vi "Check - Methods Exist.vi"(10 "QControl Class Name":string, 11 "New Class Root Path":path) -> (0 "error out":errorcluster)   [LabVIEW 2015, in "QControl Creation.lvclass"]
doc: "<b> </b> <b> </b>\n©2016 Q Software Innovations, LLC (QSI)\nwritten by Quentin Alldredge\nproduced in LabVIEW 2015\n\nsupport@qsoftwareinnovations.com\nwww.qsoftwareinnovations.com\n\nAll rights reserved.\n\nRedistribution and use in source and binary forms, with or without modification, are permitted provided that the following conditions are met:\n\n * Redistributions of source code must retain the above copyright notice, this list of conditions and the following disclaimer.\n * Redistributions in binary form must reproduce the above copyright notice, this list of conditions and the following disclaimer in the documentation and/or other materials provided with the distribution.\n * Neither the name of Q Software Innovations, LLC. nor the names of its contributors may be used to endorse or promote products derived from this software without specific prior written permission.\n\nTHIS SOFTWARE IS PROVIDED BY THE COPYRIGHT HOLDERS AND CONTRIBUTORS \"AS IS\" AND ANY EXPRESS OR IMPLIED WARRANTIES, INCLUDING, BUT NOT LIMITED TO, THE IMPLIED WARRANTIES OF MERCHANTABILITY AND FITNESS FOR A PARTICULAR PURPOSE ARE DISCLAIMED. IN NO EVENT SHALL THE COPYRIGHT OWNER OR CONTRIBUTORS BE LIABLE FOR ANY DIRECT, INDIRECT, INCIDENTAL, SPECIAL, EXEMPLARY, OR CONSEQUENTIAL DAMAGES (INCLUDING, BUT NOT LIMITED TO, PROCUREMENT OF SUBSTITUTE GOODS OR SERVICES; LOSS OF USE, DATA, OR PROFITS; OR BUSINESS INTERRUPTION) HOWEVER CAUSED AND ON ANY THEORY OF LIABILITY, WHETHER IN CONTRACT, STRICT LIABILITY, OR TORT (INCLUDING NEGLIGENCE OR OTHERWISE) ARISING IN ANY WAY OUT OF THE USE OF THIS SOFTWARE, EVEN IF ADVISED OF THE POSSIBILITY OF SUCH DAMAGE."
uses:
  QControl Creation.lvclass
  Template/Template.lvclass
  <vilib>/ErrorRing/Error Ring.xnode
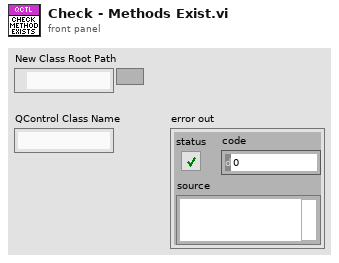
[diagram p1: front panel]
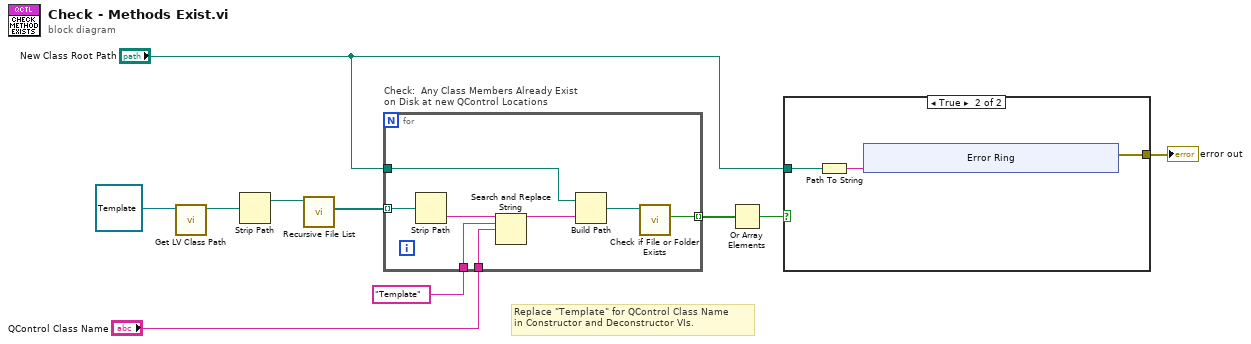
[diagram p0: block diagram]
diagram:
  # "Replace \"Template\" for QControl Class Name\nin Constructor and Deconstructor VIs."
  n1 = call <vilib>:"Get LV Class Path.vi"("object"=refnum<class "Template.lvclass"> refnum ("Template")) -> ("class path"=w8:path)  [unwired: 9 in, 1 out]
  n2 = Strip Path(path=w8) -> (stripped path=w9:path)  [unwired: 1 out]
  n3 = call <vilib>:"Recursive File List.vi"("Folder Path"=w9) -> ("All Files in Dir"=w10:path[])  [unwired: 6 in, 4 out]
  n4 = for "Check:  Any Class Members Already Exist \non Disk at new QControl Locations" {
    tunnel: w10 -> [w15] mode=indexing
    tunnel: "New Class Root Path" -> [w18]
    tunnel: [w17] -> w6 mode=indexing
    tunnel: "Template" ("search string") -> [w13]
    tunnel: "QControl Class Name" -> [w12]
    n5 = Strip Path(path=w15) -> (name=w14:string)  [unwired: 1 out]
    n6 = Search and Replace String(input string=w14, search string=w13, replace string=w12) -> (result string=w11:string)  [unwired: 5 in, 3 out]
    n7 = Build Path(base path=w18, name or relative path=w11) -> (appended path=w16:path)
    n8 = call <vilib>:"Check if File or Folder Exists.vi"("path"=w16) -> ("file or folder exists?"=w17:bool)  [unwired: 8 in, 2 out]
  }
  n9 = Or Array Elements(Boolean array=w6) -> (logical OR=w3:bool)
  n10 = case shown="True" w3 {
    tunnel: "New Class Root Path" -> [_ w21]
    tunnel: [_ w19] -> w1
    frame False {
    }
    frame True {
      n11 = Path To String(path=w21) -> (string=w20:string)
      n12 = xnode "Error Ring"("parameter 0"=w20) -> ("error out"=w19:errorcluster)
    }
  }
  "error out" <- w1
